vi "USB Open.vi"(8 "error in (no error)":errorcluster) -> (0 "error out":errorcluster, 3 "function return":i32)   [LabVIEW 2011]
uses:
  x64/Stats.lvlib
  x86/Stats32.lvlib
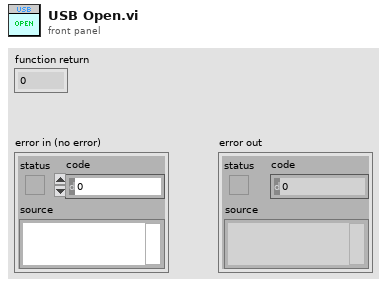
[diagram p1: front panel]
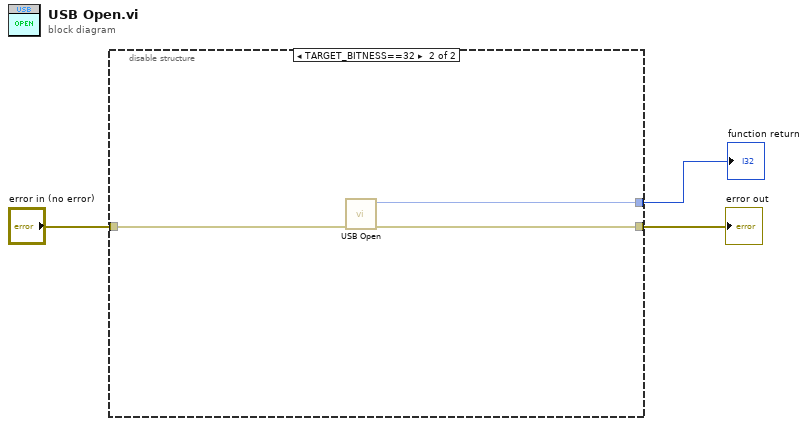
[diagram p0: block diagram]
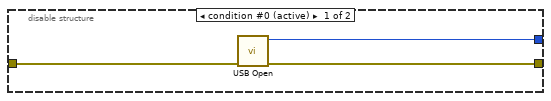
[diagram p2: hidden frame]
diagram:
  n1 = disable-structure shown="TARGET_BITNESS==32" {
    disable-tunnel: "error in (no error)" -> [w6 w7]
    disable-tunnel: [w5 w9] -> w2
    disable-tunnel: [w4 w8] -> w1
    frame condition #0 (active) {
      n2 = call "USB Open.vi"("error in (no error)"=w6) -> ("error out"=w5:errorcluster, "function return"=w4:i32)  [unwired: 9 in]
    }
    frame condition #1 {
      n3 = call "USB Open.vi"("error in (no error)"=w7) -> ("error out"=w9:errorcluster, "function return"=w8:i32)  [unwired: 9 in]
    }
  }
  "error out" <- w2
  "function return" <- w1
